vi "Event-Driven State Machine - Load Configuration.vi"() -> ()   [LabVIEW 2020]
uses:
  support/States.ctl
  support/State Machine Data.ctl
  support/Hardware Settings.ctl
  <vilib>/DAQmx/read.llb/DAQmx Read (Analog 2D DBL NChan NSamp).vi
  <vilib>/DAQmx/write.llb/DAQmx Write (Analog DBL 1Chan 1Samp).vi
  <vilib>/DAQmx/create/channels.llb/DAQmx Create Channel (AI-Voltage-Basic).vi
  <vilib>/DAQmx/configure/timing.llb/DAQmx Timing (Sample Clock).vi
  <vilib>/DAQmx/miscellaneous.llb/DAQmx Fill In Error Info.vi
  <vilib>/Utility/file.llb/Write Delimited Spreadsheet (DBL).vi
  <vilib>/DAQmx/create/channels.llb/DAQmx Create Channel (AO-Voltage-Basic).vi
panel:
  in  "Select Config File":bool
  in  "Generate Stimulus":bool
  out "RMS Results Per Channel":dbl[](array[numeric])
  out "Threshold exceeded?":bool
  in  "Acquire":bool
  in  "Threshold (rms)":dbl=1.0
  in  "Clear":bool
  in  "Exit":bool
  out "Graph":dbl[][](graph)
  # "Analysis"
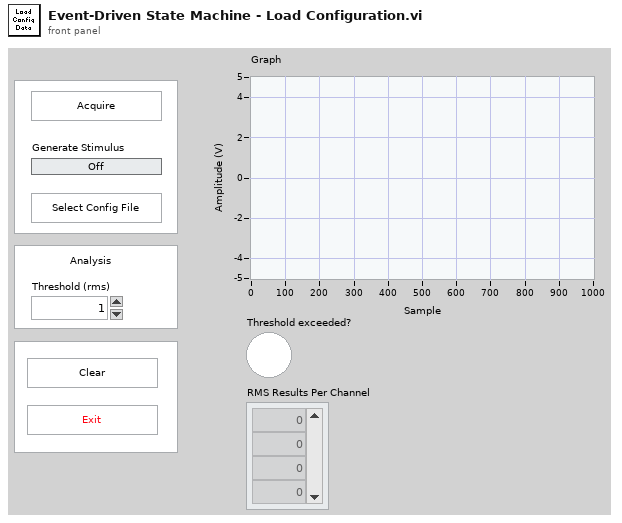
[diagram p1: front panel]
types:
  T1 = typedef "Hardware Settings.ctl" = cluster{"AI Voltage Channel":tag, "Sample Rate (Hz)":dbl, "Samples per channel":i32, "AO Voltage Channel":tag}
  T2 = typedef "State Machine Data.ctl" = cluster{"Acquisition Data":dbl[][], "Stimulus Value":bool}
  T3 = typedef "States.ctl" = enum16{"Initialize", "Wait for Event", "Acquire", "Analyze", "Log", "Clear", "Update Graph", "Update Stumulus", "Exit"}
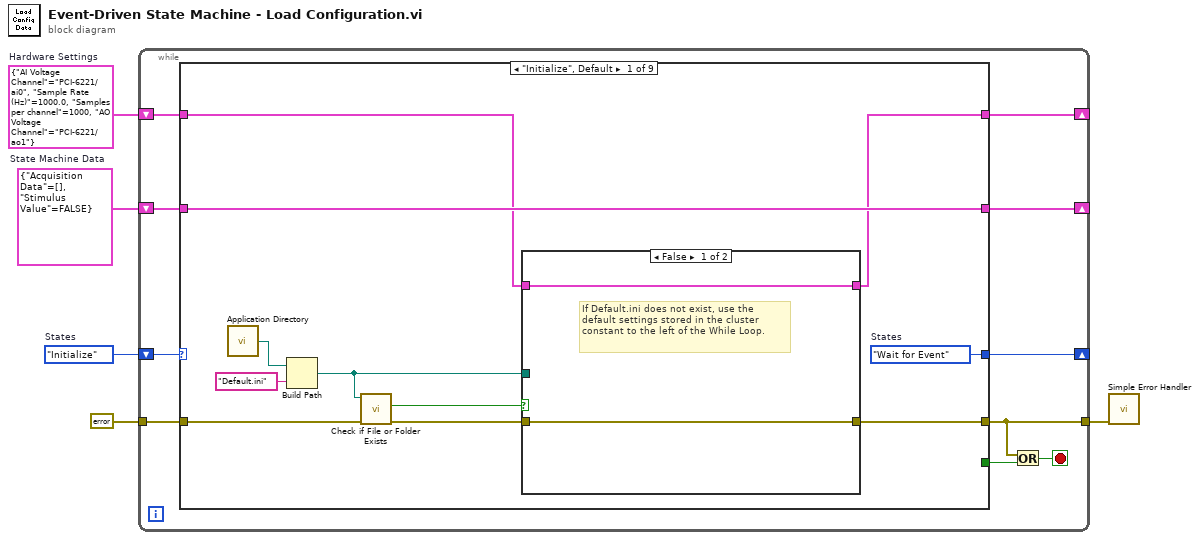
[diagram p0: block diagram]
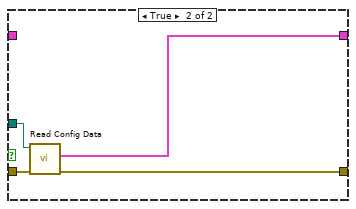
[diagram p2: hidden frame]
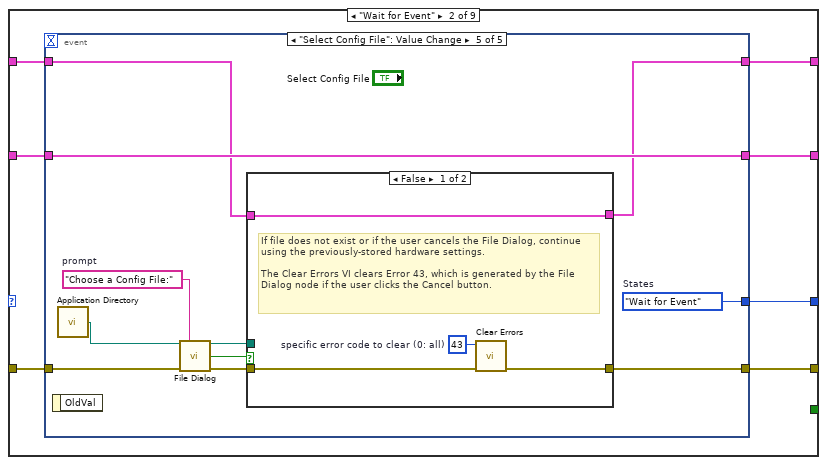
[diagram p3: hidden frame]
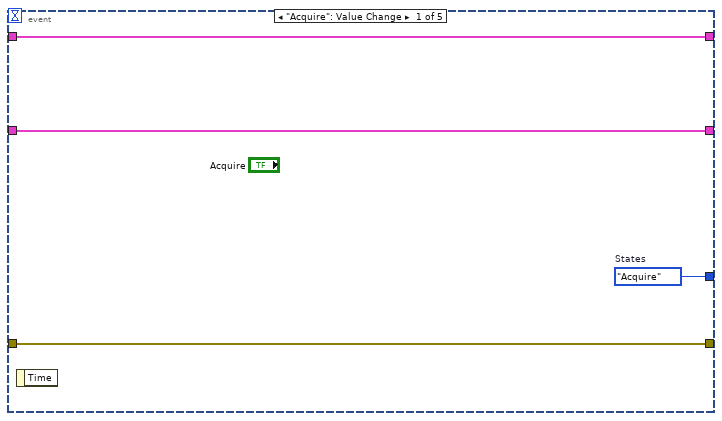
[diagram p4: hidden frame]
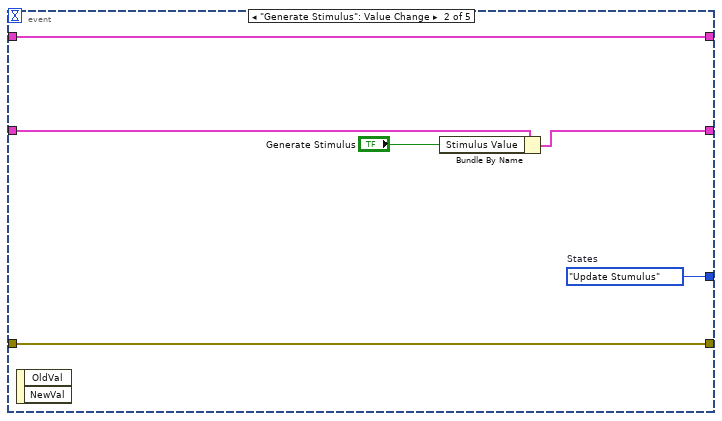
[diagram p5: hidden frame]
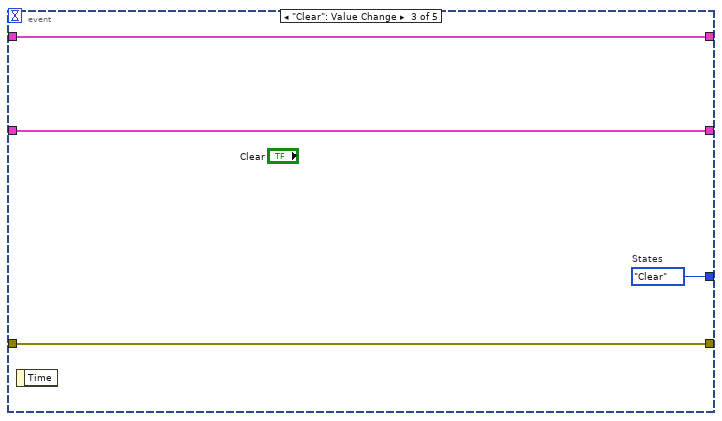
[diagram p6: hidden frame]
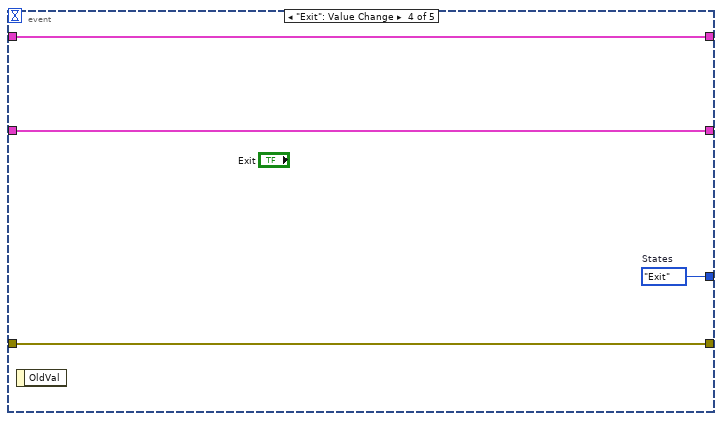
[diagram p7: hidden frame]
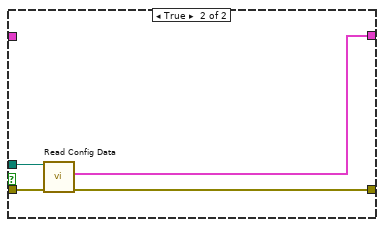
[diagram p8: hidden frame]
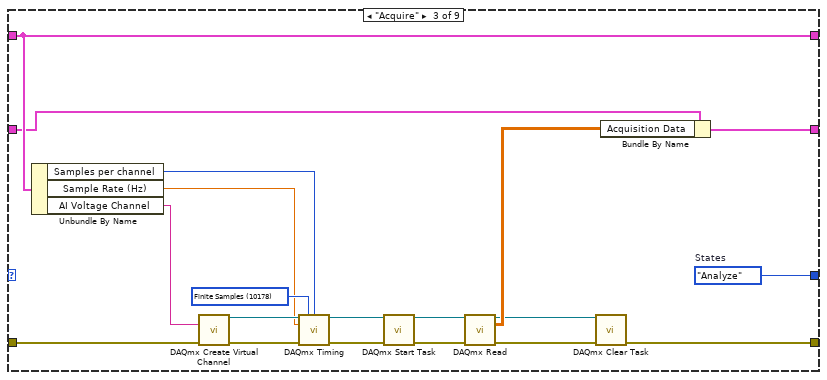
[diagram p9: hidden frame]
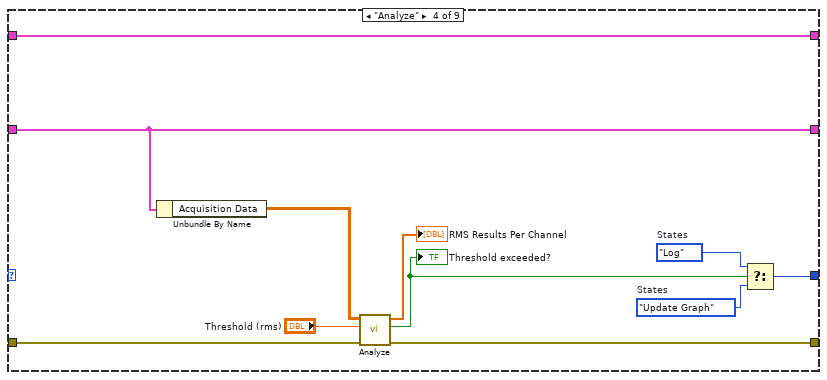
[diagram p10: hidden frame]
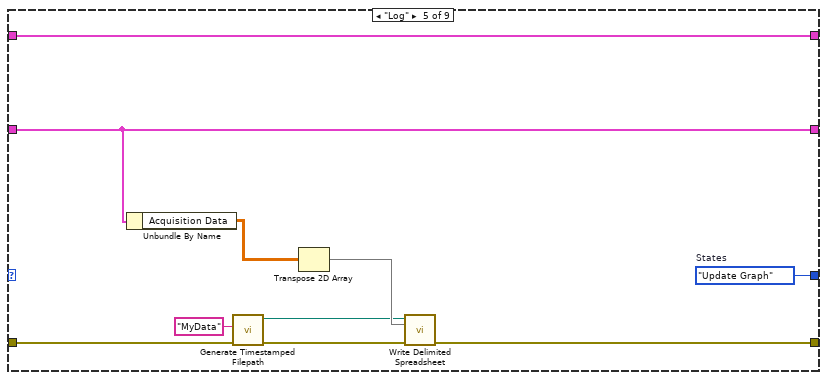
[diagram p11: hidden frame]
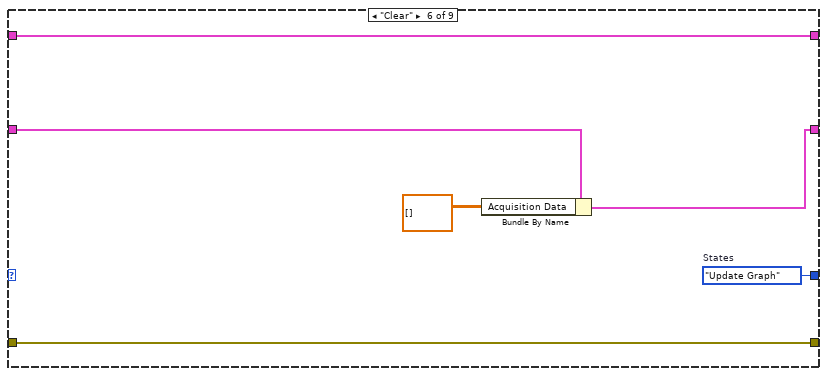
[diagram p12: hidden frame]
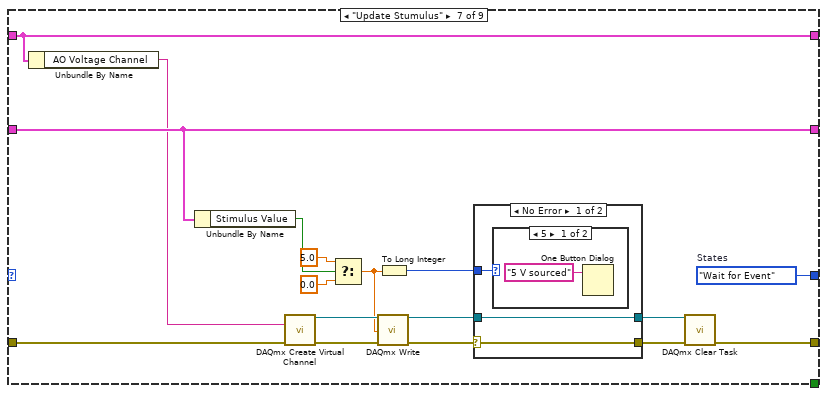
[diagram p13: hidden frame]
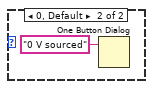
[diagram p14: hidden frame]
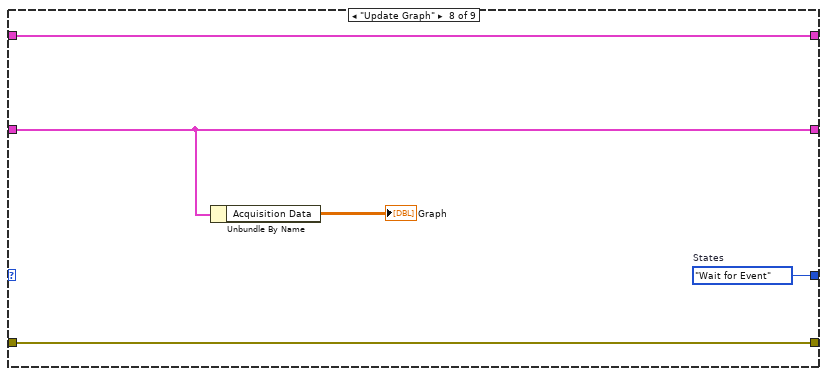
[diagram p16: hidden frame]
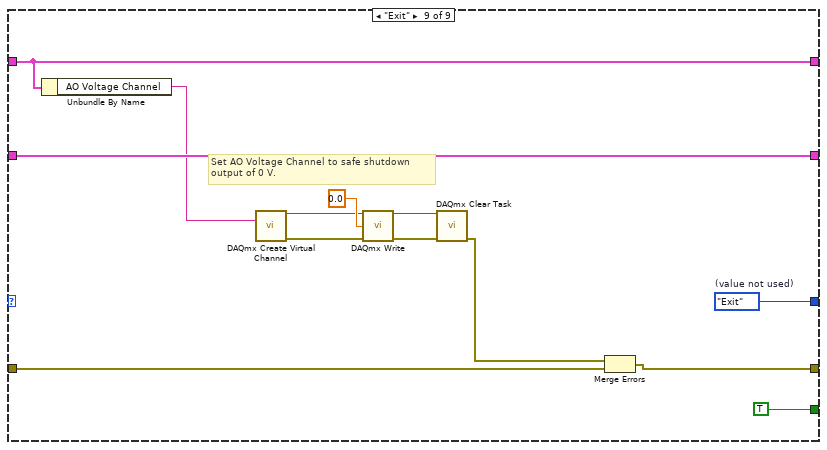
[diagram p17: hidden frame]
diagram:
  w2 = T1 {"AI Voltage Channel"="PCI-6221/ai0", "Sample Rate (Hz)"=1000.0, "Samples per channel"=1000, "AO Voltage Channel"="PCI-6221/ao1"}  # Hardware Settings
  w5 = T2 {"Acquisition Data"=[], "Stimulus Value"=FALSE}  # State Machine Data
  w4 = States."Initialize"  # States
  n1 = while {
    tunnel: errorcluster {"status"=FALSE, "code"=0, "source"=""} ("error constant") -> [w14]
    tunnel: [w10] -> w1
    shift-right: [w12] -> _
    shift-left: w5 -> [w13]
    shift-right: [w11] -> _
    shift-left: w4 -> [w15]
    shift-right: [w6] -> _
    shift-left: w2 -> [w7]
    stop <- w9 stop-if-true
    n2 = case shown="\"Initialize\", Default" w15 {
      tunnel: w14 -> [w22 w37 w95 w105 w115 w122 w130 w150 w153]
      tunnel: [w17 w36 w90 w104 w109 w122 w129 w150 w152] -> w10
      tunnel: [w26 w38 w88 w106 w116 w120 w139 w151 w164] -> w12
      tunnel: w13 -> [w26 w39 w77 w106 w116 w121 w139 w151 w164]
      tunnel: [w25 w35 w89 w100 w108 w118 w131 w149 w162] -> w11
      tunnel: [_ _ _ _ _ _ _ _ TRUE] -> w8
      tunnel: w7 -> [w18 w34 w81 w96 w107 w117 w127 w147 w161]
      tunnel: [w16 w33 w81 w96 w107 w117 w127 w147 w161] -> w6
      frame "Initialize", Default {
        w25 = States."Wait for Event"  # States
        n3 = call <vilib>:"Application Directory.vi"() -> ("Application Directory"=w24:path)
        n4 = Build Path(base path=w24, name or relative path="Default.ini") -> (appended path=w19:path)
        n5 = call <vilib>:"Check if File or Folder Exists.vi"("error in (no error)"=w22, "path"=w19) -> ("error out"=w20:errorcluster, "file or folder exists?"=w21:bool)  [unwired: 7 in, 1 out]
        n6 = case shown="False" w21 {
          tunnel: w20 -> [w27 w31]
          tunnel: w19 -> [_ w32]
          tunnel: w18 -> [w28 _]
          tunnel: [w27 w30] -> w17
          tunnel: [w28 w29] -> w16
          frame False {
            # "If Default.ini does not exist, use the default settings stored in the cluster constant to the left of the While Loop."
          }
          frame True {
            n7 = call "Read Config Data.vi"("Error In"=w31, "configuration file in"=w32) -> ("Error Out"=w30:errorcluster, "Hardware Settings"=w29:T1)  [unwired: 7 in, 1 out]
          }
        }
      }
      frame "Wait for Event" {
        n8 = event shown="[4] \"Select Config File\": Value Change" {
          selector: _ -> [_ _ _ _ _]
          dyn-events: _ -> [_ _ _ _ _]
          timeout: _ -> [_ _ _ _ _]
          tunnel: w39 -> [w43 w49 w53 w56 w68]
          tunnel: [w43 w48 w53 w56 w68] -> w38
          tunnel: w37 -> [w42 w45 w52 w57 w67]
          tunnel: [w42 w45 w52 w57 w60] -> w36
          tunnel: [w41 w46 w51 w55 w58] -> w35
          tunnel: w34 -> [w40 w44 w50 w54 w61]
          tunnel: [w40 w44 w50 w54 w59] -> w33
          event "Acquire": Value Change {
            w41 = States."Acquire"  # States
            n9 = event-data() -> ()  [unwired: 1 in, 1 out]
          }
          event "Generate Stimulus": Value Change {
            w46 = States."Update Stumulus"  # States
            n10 = event-data() -> ()  [unwired: 1 in, 2 out]
            n11 = Bundle By Name(cluster=w49, "Stimulus Value"="Generate Stimulus") -> (w48:T2)
          }
          event "Clear": Value Change {
            w51 = States."Clear"  # States
            n12 = event-data() -> ()  [unwired: 1 in, 1 out]
          }
          event "Exit": Value Change {
            w55 = States."Exit"  # States
            n13 = event-data() -> ()  [unwired: 1 in, 1 out]
          }
          event "Select Config File": Value Change {
            w58 = States."Wait for Event"  # States
            w65 = "Choose a Config File:"  # prompt
            n14 = event-data() -> ()  [unwired: 1 in, 1 out]
            n15 = call <vilib>:"Application Directory.vi"() -> ("Application Directory"=w66:path)
            n16 = call "File Dialog"("start path"=w66, "prompt"=w65, "error in"=w67) -> ("selected path"=w63:path, "exists"=w64:bool, "error out"=w62:errorcluster)  [unwired: 9 in, 1 out]
            n17 = case shown="False" w64 {
              tunnel: w63 -> [_ w76]
              tunnel: w62 -> [w70 w75]
              tunnel: w61 -> [w72 _]
              tunnel: [w69 w74] -> w60
              tunnel: [w72 w73] -> w59
              frame False {
                w71 = 43  # specific error code to clear (0: all)
                # "If file does not exist or if the user cancels the File Dialog, continue using the previously-stored hardware settings.\n\nThe Clear Errors VI clears Error 43, which is generated by the File Dialog node if the user clicks the Cancel button."
                n18 = call <vilib>:"Clear Errors.vi"("error in (no error)"=w70, "specific error code to clear (0: all)"=w71) -> ("error out"=w69:errorcluster)  [unwired: 4 in, 1 out]
              }
              frame True {
                n19 = call "Read Config Data.vi"("Error In"=w75, "configuration file in"=w76) -> ("Error Out"=w74:errorcluster, "Hardware Settings"=w73:T1)  [unwired: 7 in, 1 out]
              }
            }
          }
        }
      }
      frame "Acquire" {
        w87 = 10178 items=["Finite Samples"=10178, "Continuous Samples"=10123, "Hardware Timed Single Point"=12522] ("sample mode")
        w89 = States."Analyze"  # States
        n20 = Unbundle By Name(w81) -> ("Samples per channel"=w78:i32, "Sample Rate (Hz)"=w79:dbl, "AI Voltage Channel"=w80:tag)
        n21 = call-poly <vilib>:"DAQmx Create Virtual Channel.vi"("physical channels"=w80, "error in"=w95) -> ("task out"=w85:refnum<k21>, "error out"=w94:errorcluster)  [unwired: 12 in]
        n22 = call-poly <vilib>:"DAQmx Timing.vi"("task/channels in"=w85, "sample mode"=w87, "samples per channel"=w78, "rate"=w79, "error in"=w94) -> ("task out"=w84:refnum<k21>, "error out"=w93:errorcluster)  [unwired: 9 in]
        n23 = call <vilib>:"DAQmx Start Task.vi"("task/channels in"=w84, "error in"=w93) -> ("task out"=w83:refnum<k21>, "error out"=w92:errorcluster)  [unwired: 12 in]
        n24 = call-poly <vilib>:"DAQmx Read.vi"("task/channels in"=w83, "error in"=w92) -> ("task out"=w82:refnum<k21>, "data"=w86:dbl[][], "error out"=w91:errorcluster)  [unwired: 11 in]
        n25 = call <vilib>:"DAQmx Clear Task.vi"("task in"=w82, "error in"=w91) -> ("error out"=w90:errorcluster)  [unwired: 13 in]
        n26 = Bundle By Name(cluster=w77, "Acquisition Data"=w86) -> (w88:T2)
      }
      frame "Analyze" {
        w101 = States."Update Graph"  # States
        w102 = States."Log"  # States
        n27 = Unbundle By Name(w106) -> ("Acquisition Data"=w103:dbl[][])
        n28 = call "Analyze.vi"("Error In"=w105, "Treshold (rms)"="Threshold (rms)", "N-Channel Data (2D DBL)"=w103) -> ("Error Out"=w104:errorcluster, "Threshold exceeded?"=w97:bool, "N-Channel Data RMS Results"=→"RMS Results Per Channel":dbl[])  [unwired: 5 in, 1 out]
        "Threshold exceeded?" <- w97
        n29 = Select(t=w102, s=w97, f=w101) -> (s? t:f=w100:T3)
      }
      frame "Log" {
        w108 = States."Update Graph"  # States
        n30 = Unbundle By Name(w116) -> ("Acquisition Data"=w113:dbl[][])
        n31 = call "Generate Timestamped Filepath.vi"("Error In"=w115, "appended filename"="MyData") -> ("Error Out"=w110:errorcluster, "timestamped relative filepath"=w111:path)  [unwired: 8 in]
        n32 = Transpose 2D Array(2D array=w113) -> (transposed array=w112:dbl[][])
        n33 = call-poly <vilib>:"Write Delimited Spreadsheet.vi"("file path (dialog if empty)"=w111, "2D data"=w112, "error in (no error)"=w110) -> ("error out"=w109:errorcluster)  [unwired: 11 in, 1 out]
      }
      frame "Clear" {
        w118 = States."Update Graph"  # States
        n34 = Bundle By Name(cluster=w121, "Acquisition Data"=dbl[][] []) -> (w120:T2)
      }
      frame "Update Stumulus" {
        w131 = States."Wait for Event"  # States
        n35 = Unbundle By Name(w127) -> ("AO Voltage Channel"=w128:tag)
        n36 = Unbundle By Name(w139) -> ("Stimulus Value"=w132:bool)
        n37 = call-poly <vilib>:"DAQmx Create Virtual Channel.vi"("physical channels"=w128, "error in"=w130) -> ("task out"=w136:refnum<k21>, "error out"=w135:errorcluster)  [unwired: 12 in]
        n38 = Select(t=5.0, s=w132, f=0.0) -> (s? t:f=w134:dbl)
        n39 = call-poly <vilib>:"DAQmx Write.vi"("task/channels in"=w136, "data"=w134, "error in"=w135) -> ("task out"=w126:refnum<k21>, "error out"=w125:errorcluster)  [unwired: 10 in, 1 out]
        n40 = To Long Integer(number=w134) -> (32bit integer=w133:i32)
        n41 = case shown="No Error" w125 {
          selector: w125 -> [w140 w145]
          tunnel: w133 -> [w142 _]
          tunnel: w126 -> [w141 w146]
          tunnel: [w141 w146] -> w124
          tunnel: [w140 w145] -> w123
          frame No Error {
            n42 = case shown="5" w142 {
              frame 5 {
                n43 = One Button Dialog(message="5 V sourced") -> ()  [unwired: 1 in, 1 out]
              }
              frame 0, Default {
                n44 = One Button Dialog(message="0 V sourced") -> ()  [unwired: 1 in, 1 out]
              }
            }
          }
          frame Error {
          }
        }
        n45 = call <vilib>:"DAQmx Clear Task.vi"("task in"=w124, "error in"=w123) -> ("error out"=w129:errorcluster)  [unwired: 13 in]
      }
      frame "Update Graph" {
        w149 = States."Wait for Event"  # States
        n46 = Unbundle By Name(w151) -> ("Acquisition Data"=→"Graph":dbl[][])
      }
      frame "Exit" {
        w162 = States."Exit"  # (value not used)
        # "Set AO Voltage Channel to safe shutdown output of 0 V."
        n47 = Unbundle By Name(w161) -> ("AO Voltage Channel"=w160:tag)
        n48 = call-poly <vilib>:"DAQmx Create Virtual Channel.vi"("physical channels"=w160) -> ("task out"=w158:refnum<k21>, "error out"=w157:errorcluster)  [unwired: 13 in]
        n49 = call-poly <vilib>:"DAQmx Write.vi"("task/channels in"=w158, "data"=0.0, "error in"=w157) -> ("task out"=w155:refnum<k21>, "error out"=w156:errorcluster)  [unwired: 10 in, 1 out]
        n50 = call <vilib>:"DAQmx Clear Task.vi"("task in"=w155, "error in"=w156) -> ("error out"=w154:errorcluster)  [unwired: 13 in]
        n51 = Merge Errors(w154, w153) -> (w152:errorcluster)
      }
    }
    n52 = Or(x=w10, y=w8) -> (x .or. y?=w9:bool)
  }
  n53 = call <vilib>:"Simple Error Handler.vi"("error in (no error)"=w1) -> ()  [unwired: 4 in, 5 out]
